vi "Initialize.vi"(0 "Power Detector in":refnum<class "Power Detector.lvclass">, 11 "error in":errorcluster) -> (4 "Power Detector out":refnum<class "Power Detector.lvclass">, 15 "error out":errorcluster)   [LabVIEW 2023, in "NI CAL-5501 Power Detector.lvlib" / "Power Detector.lvclass"]
uses:
  Power Detector.lvclass
  C:/srd-semi-rfcal-software/AuxTools/STSRFFixtureCharactUtility/Source/Code Modules/Fixture/Instruments/Power Meter/Power Meter Base/Power Meter Base.lvclass
  Instruments/Power Meter/Power Meter Base/Power Meter Base.lvclass/Power Meter Base.ctl
  Power Detector.lvclass/Power Detector.ctl
  Instruments/Power Meter/Power Meter Base/Properties/Read Active Instrument Info.vi
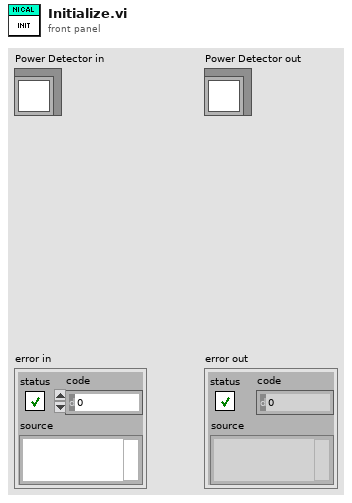
[diagram p1: front panel]
types:
  T1 = typedef "RFFixtureCharact.Instruments.lvlib/Power Meter Base.lvclass/Instrument Info.ctl" = cluster{"User Alias":string, "Resource Name":string, "Product Name":string, "Vendor Name":string}
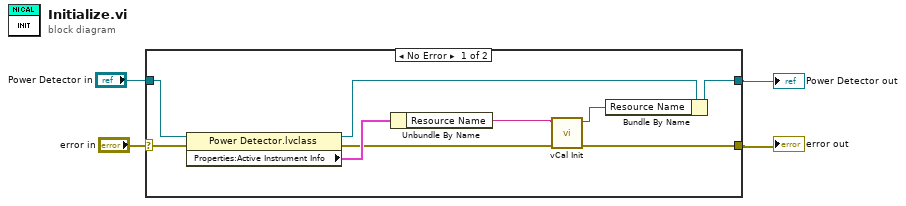
[diagram p0: block diagram]
diagram:
  n1 = case shown="No Error" "error in" {
    selector: "error in" -> [w13 w15]
    tunnel: [w8 w15] -> w3
    tunnel: "Power Detector in" -> [w12 w14]
    tunnel: [w7 w14] -> w1
    frame No Error {
      n2 = property class="Power Detector.lvclass"(reference=w12, error in=w13) -> (reference out=w11:refnum<class "Power Detector.lvclass">, error out=w9:errorcluster, "Properties:Active Instrument Info"=w10:T1)
      n3 = Unbundle By Name(w10) -> ("Resource Name"=w6:string)
      n4 = call <instrlib>:"vCal Init.vi"("error in"=w9, "resource name"=w6) -> ("error out"=w8:errorcluster, "instrument handle"=w5:refnum<k15>)  [unwired: 8 in]
      n5 = Bundle By Name(cluster=w11, "Resource Name"=w5) -> (w7:refnum<class "Power Detector.lvclass">)
    }
    frame Error {
    }
  }
  "error out" <- w3
  "Power Detector out" <- w1
